vi "获取控制器信息.vi"(8 "error in (no error)":errorcluster, 11 "MB session in":refnum<class "MB_Master.lvclass">) -> (0 "error out":errorcluster, 2 "控制器信息":cluster{"设备温度℃":dbl}, 3 "MB session out":refnum<class "MB_Master.lvclass">)   [LabVIEW 2016, in "环境动力单元.lvlib"]
uses:
  <vilib>/Plasmionique/MB Master/MB_Master/MB_Master.lvclass
  <vilib>/Plasmionique/MB Master/MB Master.lvlib
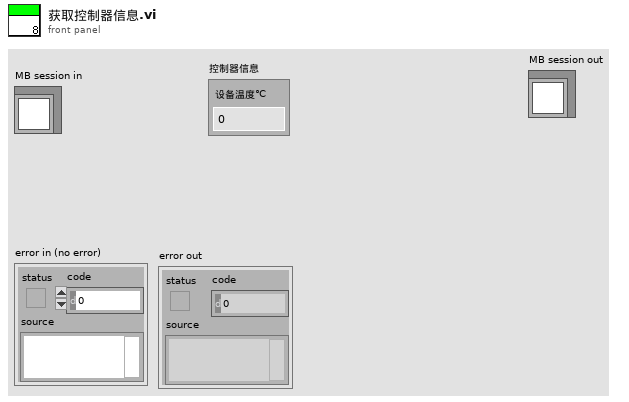
[diagram p1: front panel]
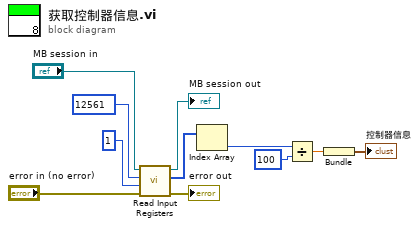
[diagram p0: block diagram]
diagram:
  n1 = call <vilib>:"Read Input Registers.vi"("error in (no error)"="error in (no error)", "quantity"=u16 1, "starting address"=u16 12561, "MB session in"="MB session in") -> ("error out"=→"error out":errorcluster, "Registers"=w7:u16[], "MB session out"=→"MB session out":refnum<class "MB_Master.lvclass">)  [unwired: 5 in]
  n2 = Index Array(array=w7) -> (element=w6:u16)  [unwired: 1 in]
  n3 = Divide(x=w6, y=u16 100) -> (x/y=w4:dbl)
  n4 = Bundle(w4) -> (→"控制器信息":cluster{dbl})  [unwired: 1 in]
